vi "WSVCAP SHL FPGA LL I2C Write CLK or DATA Lines.vi"(0 "Bit In":bool, 11 "error in (no error)":errorcluster, 13 "Line":T1, 14 "Socket Mask":u64 format="%08x") -> (15 "error out":errorcluster)   [LabVIEW 2012]
uses:
  Type Defs/WSVCAP SHL I2C Write Line Enum.ctl
  <vilib>/rvi/eio/common/nirviEmuTemplateMethod_errors.vi
  <vilib>/eio/EIONode/EIONode.xnode
  WSVCAP SHL FPGA LL I2C Debug Global.vi
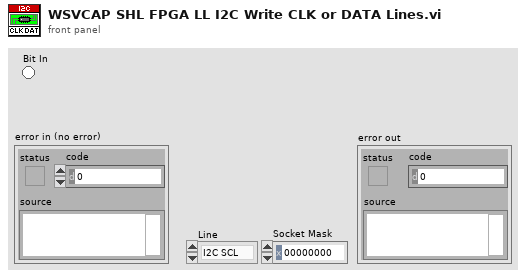
[diagram p1: front panel]
types:
  T1 = typedef "WSVCAP SHL I2C Write Line Enum.ctl" = enum16{"I2C SCL", "I2C SDA"}
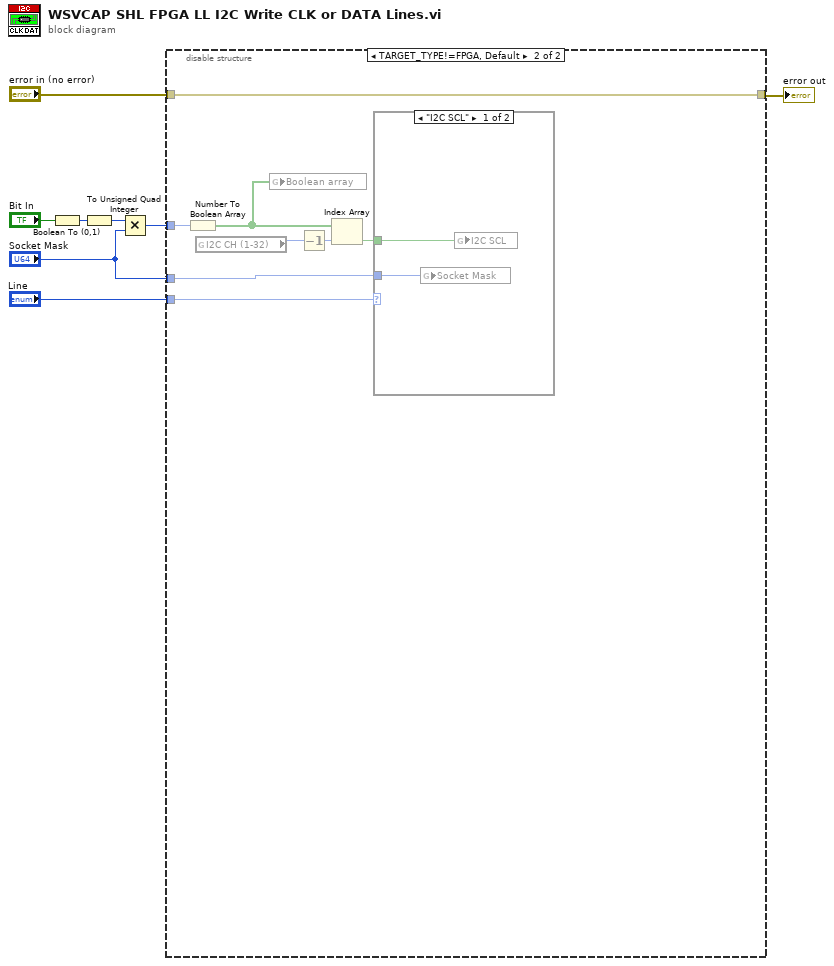
[diagram p0: block diagram]
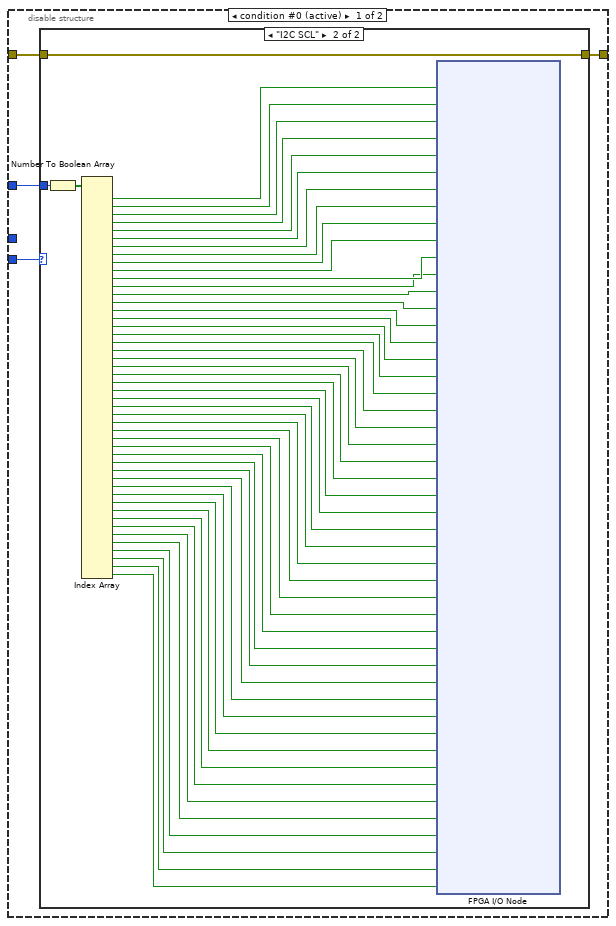
[diagram p2: hidden frame]
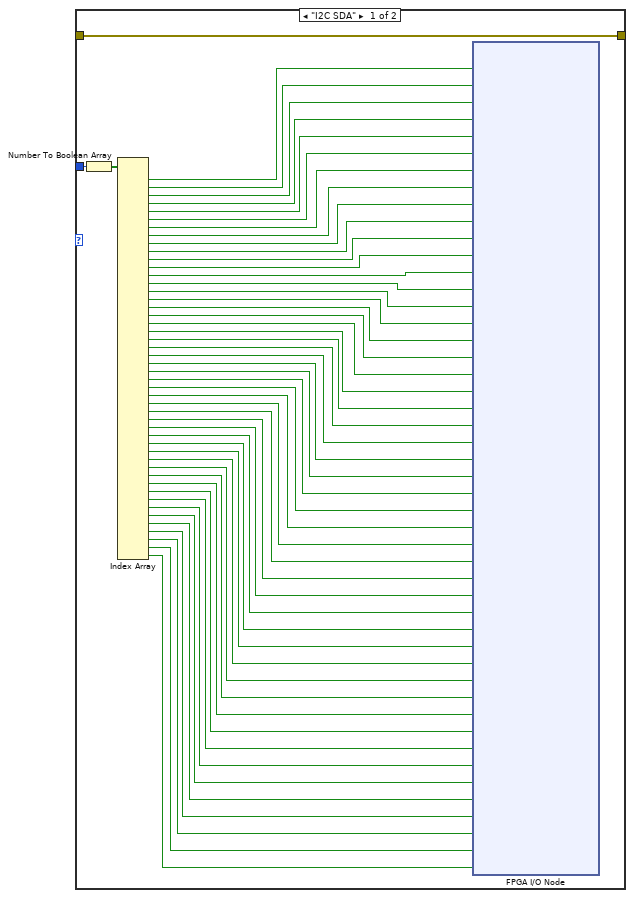
[diagram p3: hidden frame]
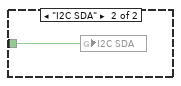
[diagram p4: hidden frame]
diagram:
  n1 = Boolean To (0,1)(Boolean="Bit In") -> (0, 1=w5:i16)
  n2 = To Unsigned Quad Integer(1:w5) -> (0:w4:u64)
  n3 = Multiply(x=w4, y="Socket Mask") -> (x*y=w2:u64)
  n4 = disable-structure shown="TARGET_TYPE!=FPGA, Default" {
    disable-tunnel: w2 -> [w12 w117]
    disable-tunnel: "Line" -> [w11 w122]
    disable-tunnel: [w10 w121] -> w7
    disable-tunnel: "error in (no error)" -> [w9 w121]
    disable-tunnel: "Socket Mask" -> [_ w115]
    frame condition #0 (active) {
      n5 = case shown="\"I2C SCL\"" w11 {
        tunnel: w12 -> [w62 w113]
        tunnel: [w29 w80] -> w10
        tunnel: w9 -> [w29 w80]
        frame "I2C SDA" {
          n6 = Number To Boolean Array(number=w62) -> (Boolean array=w63:bool[])
          n7 = Index Array(array=w63) -> (element #1=w61:bool, element #2=w60:bool, element #3=w59:bool, element #4=w58:bool, element #5=w57:bool, element #6=w56:bool, element #7=w55:bool, element #8=w54:bool, element #9=w53:bool, element #10=w52:bool, element #11=w51:bool, element #12=w50:bool, element #13=w49:bool, element #14=w48:bool, element #15=w47:bool, element #16=w46:bool, element #17=w45:bool, element #18=w44:bool, element #19=w43:bool, element #20=w42:bool, element #21=w41:bool, element #22=w40:bool, element #23=w39:bool, element #24=w38:bool, element #25=w37:bool, element #26=w36:bool, element #27=w35:bool, element #28=w34:bool, element #29=w33:bool, element #30=w32:bool, element #31=w31:bool, element #32=w30:bool, element #33=w28:bool, element #34=w27:bool, element #35=w26:bool, element #36=w25:bool, element #37=w24:bool, element #38=w23:bool, element #39=w22:bool, element #40=w21:bool, element #41=w20:bool, element #42=w19:bool, element #43=w18:bool, element #44=w17:bool, element #45=w16:bool, element #46=w15:bool, element #47=w14:bool, element #48=w13:bool)  [unwired: 48 in]
          n8 = xnode "FPGA I/O Node"("I2C_SDA_C1_S1"=w61, "I2C_SDA_C1_S2"=w60, "I2C_SDA_C1_S3"=w59, "I2C_SDA_C1_S4"=w58, "I2C_SDA_C1_S5"=w57, "I2C_SDA_C1_S6"=w56, "I2C_SDA_C1_S7"=w55, "I2C_SDA_C1_S8"=w54, "I2C_SDA_C1_S9"=w53, "I2C_SDA_C1_S10"=w52, "I2C_SDA_C1_S11"=w51, "I2C_SDA_C1_S12"=w50, "I2C_SDA_C1_S13"=w49, "I2C_SDA_C1_S14"=w48, "I2C_SDA_C1_S15"=w47, "I2C_SDA_C1_S16"=w46, "I2C_SDA_C2_S1"=w45, "I2C_SDA_C2_S2"=w44, "I2C_SDA_C2_S3"=w43, "I2C_SDA_C2_S4"=w42, "I2C_SDA_C2_S5"=w41, "I2C_SDA_C2_S6"=w40, "I2C_SDA_C2_S7"=w39, "I2C_SDA_C2_S8"=w38, "I2C_SDA_C2_S9"=w37, "I2C_SDA_C2_S10"=w36, "I2C_SDA_C2_S11"=w35, "I2C_SDA_C2_S12"=w34, "I2C_SDA_C2_S13"=w33, "I2C_SDA_C2_S14"=w32, "I2C_SDA_C2_S15"=w31, "I2C_SDA_C2_S16"=w30, "I2C_SDA_C3_S1"=w28, "I2C_SDA_C3_S2"=w27, "I2C_SDA_C3_S3"=w26, "I2C_SDA_C3_S4"=w25, "I2C_SDA_C3_S5"=w24, "I2C_SDA_C3_S6"=w23, "I2C_SDA_C3_S7"=w22, "I2C_SDA_C3_S8"=w21, "I2C_SDA_C3_S9"=w20, "I2C_SDA_C3_S10"=w19, "I2C_SDA_C3_S11"=w18, "I2C_SDA_C3_S12"=w17, "I2C_SDA_C3_S13"=w16, "I2C_SDA_C3_S14"=w15, "I2C_SDA_C3_S15"=w14, "I2C_SDA_C3_S16"=w13) -> ()  [unwired: 48 in, 48 out]
        }
        frame "I2C SCL" {
          n9 = Number To Boolean Array(number=w113) -> (Boolean array=w114:bool[])
          n10 = Index Array(array=w114) -> (element #1=w112:bool, element #2=w111:bool, element #3=w110:bool, element #4=w109:bool, element #5=w108:bool, element #6=w107:bool, element #7=w106:bool, element #8=w105:bool, element #9=w104:bool, element #10=w103:bool, element #11=w102:bool, element #12=w101:bool, element #13=w100:bool, element #14=w99:bool, element #15=w98:bool, element #16=w97:bool, element #17=w96:bool, element #18=w95:bool, element #19=w94:bool, element #20=w93:bool, element #21=w92:bool, element #22=w91:bool, element #23=w90:bool, element #24=w89:bool, element #25=w88:bool, element #26=w87:bool, element #27=w86:bool, element #28=w85:bool, element #29=w84:bool, element #30=w83:bool, element #31=w82:bool, element #32=w81:bool, element #33=w79:bool, element #34=w78:bool, element #35=w77:bool, element #36=w76:bool, element #37=w75:bool, element #38=w74:bool, element #39=w73:bool, element #40=w72:bool, element #41=w71:bool, element #42=w70:bool, element #43=w69:bool, element #44=w68:bool, element #45=w67:bool, element #46=w66:bool, element #47=w65:bool, element #48=w64:bool)  [unwired: 48 in]
          n11 = xnode "FPGA I/O Node"("I2C_SCL_C1_S1"=w112, "I2C_SCL_C1_S2"=w111, "I2C_SCL_C1_S3"=w110, "I2C_SCL_C1_S4"=w109, "I2C_SCL_C1_S5"=w108, "I2C_SCL_C1_S6"=w107, "I2C_SCL_C1_S7"=w106, "I2C_SCL_C1_S8"=w105, "I2C_SCL_C1_S9"=w104, "I2C_SCL_C1_S10"=w103, "I2C_SCL_C1_S11"=w102, "I2C_SCL_C1_S12"=w101, "I2C_SCL_C1_S13"=w100, "I2C_SCL_C1_S14"=w99, "I2C_SCL_C1_S15"=w98, "I2C_SCL_C1_S16"=w97, "I2C_SCL_C2_S1"=w96, "I2C_SCL_C2_S2"=w95, "I2C_SCL_C2_S3"=w94, "I2C_SCL_C2_S4"=w93, "I2C_SCL_C2_S5"=w92, "I2C_SCL_C2_S6"=w91, "I2C_SCL_C2_S7"=w90, "I2C_SCL_C2_S8"=w89, "I2C_SCL_C2_S9"=w88, "I2C_SCL_C2_S10"=w87, "I2C_SCL_C2_S11"=w86, "I2C_SCL_C2_S12"=w85, "I2C_SCL_C2_S13"=w84, "I2C_SCL_C2_S14"=w83, "I2C_SCL_C2_S15"=w82, "I2C_SCL_C2_S16"=w81, "I2C_SCL_C3_S1"=w79, "I2C_SCL_C3_S2"=w78, "I2C_SCL_C3_S3"=w77, "I2C_SCL_C3_S4"=w76, "I2C_SCL_C3_S5"=w75, "I2C_SCL_C3_S6"=w74, "I2C_SCL_C3_S7"=w73, "I2C_SCL_C3_S8"=w72, "I2C_SCL_C3_S9"=w71, "I2C_SCL_C3_S10"=w70, "I2C_SCL_C3_S11"=w69, "I2C_SCL_C3_S12"=w68, "I2C_SCL_C3_S13"=w67, "I2C_SCL_C3_S14"=w66, "I2C_SCL_C3_S15"=w65, "I2C_SCL_C3_S16"=w64) -> ()  [unwired: 48 in, 48 out]
        }
      }
    }
    frame condition #1 {
      n12 = Number To Boolean Array(number=w117) -> (Boolean array=w116:bool[])
      n13 = global read "WSVCAP SHL FPGA LL I2C Debug Global.vi" "I2C CH (1-32)"() -> (w119:i32)
      n14 = global write "WSVCAP SHL FPGA LL I2C Debug Global.vi" "Boolean array"(w116) -> ()
      n15 = Decrement(x=w119) -> (x-1=w118:i32)
      n16 = Index Array(array=w116, index=w118) -> (element=w120:bool)
      n17 = case shown="\"I2C SCL\"" w122 {
        tunnel: w120 -> [w124 w125]
        tunnel: w115 -> [w123 _]
        frame "I2C SCL" {
          n18 = global write "WSVCAP SHL FPGA LL I2C Debug Global.vi" "Socket Mask"(w123) -> ()
          n19 = global write "WSVCAP SHL FPGA LL I2C Debug Global.vi" "I2C SCL"(w124) -> ()
        }
        frame "I2C SDA" {
          n20 = global write "WSVCAP SHL FPGA LL I2C Debug Global.vi" "I2C SDA"(w125) -> ()
        }
      }
    }
  }
  "error out" <- w7
